vi "Sample preparation.vi"(6 "ALS mode parameter":T1={"Wash vial Location"=0.0, "Reagent volume (ul)"=[], "Reagent location"=[], "Mix vial Location"=0.0, "Pump 5 target volume (ml)"=5.0, "Pump 5  flowrate (ml/min)"=5.0, "Sample name"=""} {"Pump 5  flowrate (ml/min)" min=0.0 format="%#.4f"; "Pump 5 target volume (ml)" min=0.0 format="%#.4f"}, 7 "Syringe mode parameter":T2={"Pump 5 charge rate (ml/min)"=0.5, "Pump 5 charge volume (mL)"=0.1} {"Pump 5 charge volume (mL)" format="%#.4f"; "Pump 5 charge rate (ml/min)" format="%#.4f"}, 8 "Sample source":enum16{"Syringe", "ALS"}(ring), 9 "Experiment file path":path, 10 "Method folder":path=path "\\\\ECHEMHPLC-PC\\Chem32(2)/1/Data/OptSys.D", 11 "Configured COM ports":T3={"Pump 1 COM"="COM12", "Pump 2 COM"="COM9", "Pump 3 COM"="COM13", "Pump 4 COM"="COM4", "Pump 5 COM"="COM15"}) -> ()   [LabVIEW 2017]
uses:
  <instrlib>/Harvard Apparatus PHD Ultra Series/Harvard Apparatus PHD Ultra Series.lvlib
panel:
  out "ALS droplet time":string
  out "Pump 5 COM":refnum<visa-resource-name>="COM12"
  out "Pump 1 COM":refnum<visa-resource-name>="COM12"
  out "Pump 2 COM":refnum<visa-resource-name>="COM12"
  out "Pump 3 COM":refnum<visa-resource-name>="COM12"
  out "Pump 4 COM":refnum<visa-resource-name>="COM12"
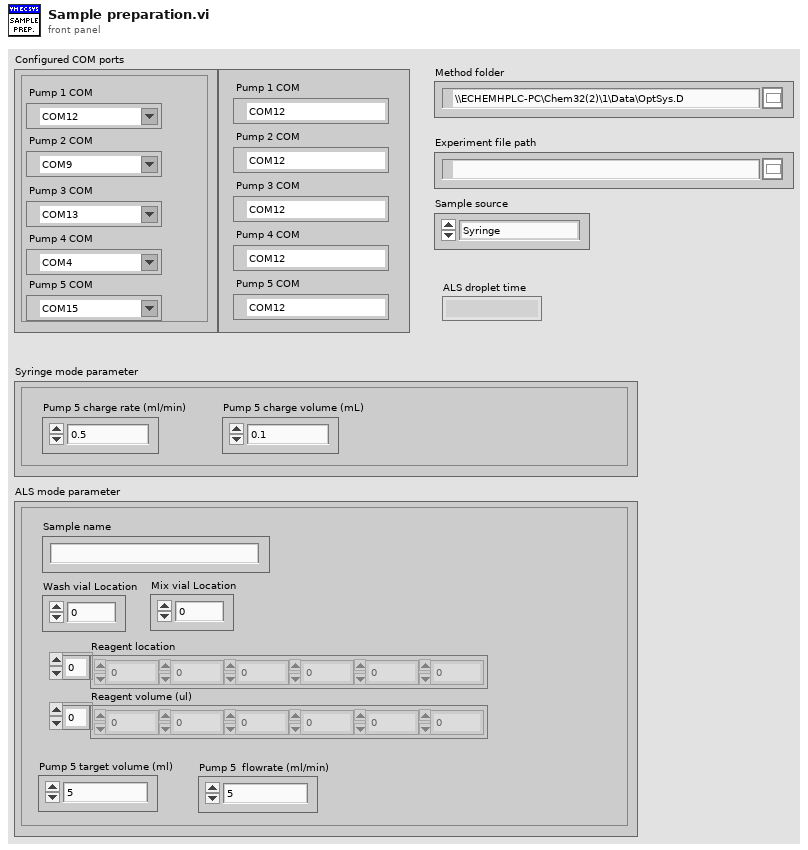
[diagram p1: front panel]
types:
  T1 = cluster{"Wash vial Location":dbl, "Reagent volume (ul)":dbl[], "Reagent location":dbl[], "Mix vial Location":dbl, "Pump 5 target volume (ml)":dbl, "Pump 5  flowrate (ml/min)":dbl, "Sample name":string}
  T2 = cluster{"Pump 5 charge rate (ml/min)":dbl, "Pump 5 charge volume (mL)":dbl}
  T3 = cluster{"Pump 1 COM":refnum<visa-resource-name>, "Pump 2 COM":refnum<visa-resource-name>, "Pump 3 COM":refnum<visa-resource-name>, "Pump 4 COM":refnum<visa-resource-name>, "Pump 5 COM":refnum<visa-resource-name>}
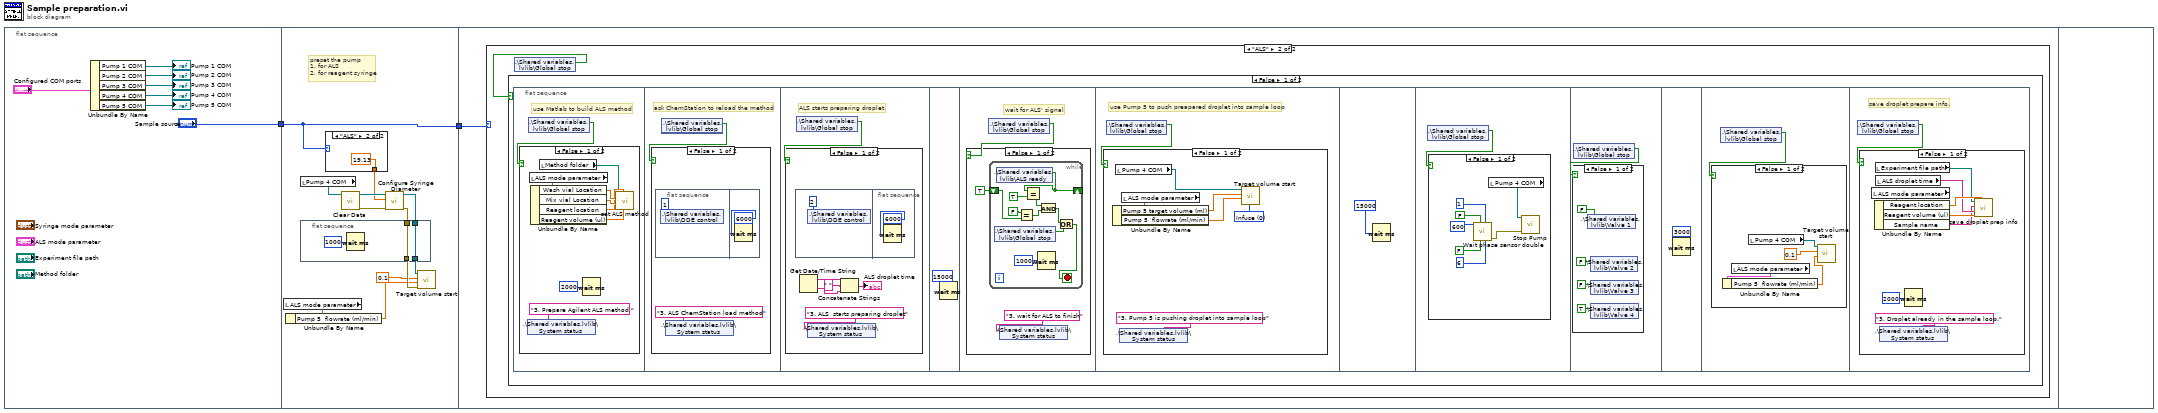
[diagram p0: block diagram]
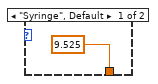
[diagram p2: hidden frame]
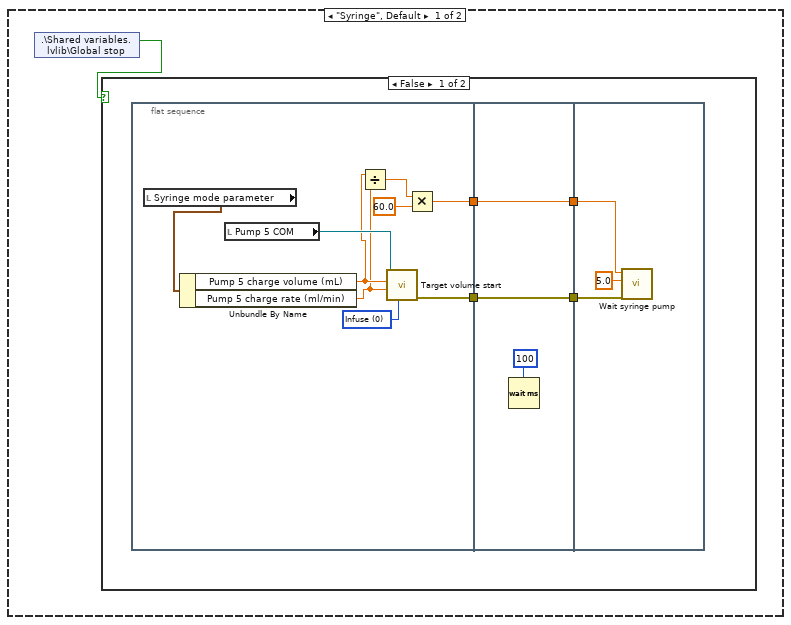
[diagram p3: hidden frame]
diagram:
  n1 = flat-sequence {
    tunnel: ["Sample source"] -> w2
    tunnel: w2 -> [w17]
    tunnel: [w17] -> w1
    tunnel: w1 -> [w27]
    frame #0 {
      n2 = Unbundle By Name("Configured COM ports") -> ("Pump 1 COM"=→"Pump 1 COM":refnum<visa-resource-name>, "Pump 2 COM"=→"Pump 2 COM":refnum<visa-resource-name>, "Pump 3 COM"=→"Pump 3 COM":refnum<visa-resource-name>, "Pump 4 COM"=→"Pump 4 COM":refnum<visa-resource-name>, "Pump 5 COM"=→"Pump 5 COM":refnum<visa-resource-name>)
    }
    frame #1 {
      # "preset the pump\n1. for ALS\n2. for reagent syringe"
      n3 = local read "ALS mode parameter"() -> (w12:T1)
      n4 = Unbundle By Name(w12) -> ("Pump 5  flowrate (ml/min)"=w11:dbl)
      n5 = local read "Pump 4 COM"() -> (w18:refnum<visa-resource-name>)
      n6 = flat-sequence {
        tunnel: [w23] -> w16
        tunnel: w15 -> [w23]
        tunnel: [w22] -> w14
        tunnel: w13 -> [w22]
        frame #0 {
          n7 = Wait (ms)(milliseconds to wait=u32 1000) -> ()  [unwired: 1 out]
        }
      }
      n8 = case shown="\"ALS\"" w17 {
        tunnel: [9.525 ("Syringe Diameter (20 mm)") 19.13 ("Syringe Diameter (20 mm)")] -> w19
        frame "Syringe", Default {
        }
        frame "ALS" {
        }
      }
      n9 = call <instrlib>:"Clear Data.vi"("VISA resource name"=w18) -> ("error out"=w21:errorcluster, "VISA resource name out"=w20:refnum<visa-resource-name>)  [unwired: 9 in]
      n10 = call <instrlib>:"Configure Syringe Diameter.vi"("error in (no error)"=w21, "Syringe Diameter (20 mm)"=w19, "VISA resource name"=w20) -> ("error out"=w15:errorcluster, "VISA resource name out"=w13:refnum<visa-resource-name>)  [unwired: 7 in]
      n11 = call "Target volume start.vi"("error in (no error)"=w16, "Flow Rate (ml/min)"=w11, "Target volume (ml)"=0.1, "VISA resource name"=w14) -> ()  [unwired: 6 in, 2 out]
    }
    frame #2 {
      n12 = case shown="\"ALS\"" w27 {
        frame "Syringe", Default {
          n13 = shared-variable ".\\Shared variables.lvlib\\Global stop"() -> (w28:bool)  [unwired: 1 in, 1 out]
          n14 = case shown="False" w28 {
            frame False {
              n15 = flat-sequence {
                tunnel: [w39] -> w32
                tunnel: [w36] -> w31
                tunnel: [w43] -> w30
                tunnel: w32 -> [w43]
                tunnel: [w42] -> w29
                tunnel: w31 -> [w42]
                tunnel: w30 -> [w47]
                tunnel: w29 -> [w45]
                frame #0 {
                  w40 = u16 0 items=["Infuse", "Withdraw"] ("Pump Direction (0:Infuse)")
                  n16 = local read "Syringe mode parameter"() -> (w35:T2)
                  n17 = Unbundle By Name(w35) -> ("Pump 5 charge volume (mL)"=w34:dbl, "Pump 5 charge rate (ml/min)"=w33:dbl)
                  n18 = local read "Pump 5 COM"() -> (w41:refnum<visa-resource-name>)
                  n19 = Divide(x=w34, y=w33) -> (x/y=w38:dbl)
                  n20 = call "Target volume start.vi"("Pump Direction (0:Infuse)"=w40, "Flow Rate (ml/min)"=w33, "Target volume (ml)"=w34, "VISA resource name"=w41) -> ("error out"=w39:errorcluster)  [unwired: 6 in, 1 out]
                  n21 = Multiply(x=w38, y=60.0) -> (x*y=w36:dbl)
                }
                frame #1 {
                  n22 = Wait (ms)(milliseconds to wait=u32 100) -> ()  [unwired: 1 out]
                }
                frame #2 {
                  n23 = call "Wait syringe pump.vi"("error in (no error)"=w47, "Delayed time (s)"=5.0, "Time Target (s)"=w45) -> ()  [unwired: 8 in, 1 out]
                }
              }
            }
            frame True {
            }
          }
        }
        frame "ALS" {
          n24 = shared-variable ".\\Shared variables.lvlib\\Global stop"() -> (w48:bool)  [unwired: 1 in, 1 out]
          n25 = case shown="False" w48 {
            frame False {
              n26 = flat-sequence {
                frame #0 {
                  # "use Matlab to build ALS method"
                  n27 = shared-variable ".\\Shared variables.lvlib\\Global stop"() -> (w49:bool)  [unwired: 1 in, 1 out]
                  n28 = case shown="False" w49 {
                    frame False {
                      n29 = shared-variable ".\\Shared variables.lvlib\\System status"("3. Prepare Agilent ALS method " ("System status")) -> ()  [unwired: 1 in, 1 out]
                      n30 = local read "ALS mode parameter"() -> (w56:T1)
                      n31 = Unbundle By Name(w56) -> ("Wash vial Location"=w55:dbl, "Mix vial Location"=w54:dbl, "Reagent location"=w52:dbl[], "Reagent volume (ul)"=w53:dbl[])
                      n32 = local read "Method folder"() -> (w51:path)
                      n33 = Wait (ms)(milliseconds to wait=u32 2000) -> ()  [unwired: 1 out]
                      n34 = call "set ALS method.vi"("Reagent volume (ul)"=w53, "Reagent location"=w52, "Mix vial Location"=w54, "Wash vial Location"=w55, "method folder"=w51) -> ()  [unwired: 7 in]
                    }
                    frame True {
                    }
                  }
                }
                frame #1 {
                  # "ask ChemStation to reload the method"
                  n35 = shared-variable ".\\Shared variables.lvlib\\Global stop"() -> (w58:bool)  [unwired: 1 in, 1 out]
                  n36 = case shown="False" w58 {
                    frame False {
                      n37 = flat-sequence {
                        frame #0 {
                          n38 = shared-variable ".\\Shared variables.lvlib\\DDE control"(i8 1 ("DDE control")) -> ()  [unwired: 1 in, 1 out]
                        }
                        frame #1 {
                          n39 = Wait (ms)(milliseconds to wait=u32 6000) -> ()  [unwired: 1 out]
                        }
                      }
                      n40 = shared-variable ".\\Shared variables.lvlib\\System status"("3. ALS ChemStation load method" ("System status")) -> ()  [unwired: 1 in, 1 out]
                    }
                    frame True {
                    }
                  }
                  n41 = shared-variable ".\\Shared variables.lvlib\\Global stop"() -> ()  [unwired: 1 in, 2 out]
                }
                frame #2 {
                  # "ALS starts preparing droplet"
                  n42 = shared-variable ".\\Shared variables.lvlib\\Global stop"() -> (w62:bool)  [unwired: 1 in, 1 out]
                  n43 = case shown="False" w62 {
                    frame False {
                      n44 = flat-sequence {
                        frame #0 {
                          n45 = shared-variable ".\\Shared variables.lvlib\\DDE control"(i8 2 ("DDE control")) -> ()  [unwired: 1 in, 1 out]
                        }
                        frame #1 {
                          n46 = Wait (ms)(milliseconds to wait=u32 6000) -> ()  [unwired: 1 out]
                        }
                      }
                      n47 = Get Date/Time String() -> (date string=w66:string, time string=w64:string)  [unwired: 3 in]
                      n48 = shared-variable ".\\Shared variables.lvlib\\System status"("3. ALS  starts preparing droplet" ("System status")) -> ()  [unwired: 1 in, 1 out]
                      n49 = Concatenate Strings(w66, " ", w64) -> (→"ALS droplet time":string)
                    }
                    frame True {
                    }
                  }
                }
                frame #3 {
                  n50 = Wait (ms)(milliseconds to wait=u32 15000) -> ()  [unwired: 1 out]
                }
                frame #4 {
                  # "wait for ALS' signal"
                  n51 = shared-variable ".\\Shared variables.lvlib\\Global stop"() -> (w71:bool)  [unwired: 1 in, 1 out]
                  n52 = case shown="False" w71 {
                    frame False {
                      n53 = while {
                        shift-right: [w80] -> _
                        shift-left: TRUE ("Boolean") -> [w79]
                        stop <- w82 stop-if-true
                        n54 = shared-variable ".\\Shared variables.lvlib\\Global stop"() -> (w83:bool)  [unwired: 1 in, 1 out]
                        n55 = shared-variable ".\\Shared variables.lvlib\\ALS ready"() -> (w80:bool)  [unwired: 1 in, 1 out]
                        n56 = Equal?(x=FALSE, y=w79) -> (x = y?=w75:bool)
                        n57 = Equal?(x=w80, y=TRUE) -> (x = y?=w76:bool)
                        n58 = Wait (ms)(milliseconds to wait=u32 1000) -> ()  [unwired: 1 out]
                        n59 = And(x=w76, y=w75) -> (x .and. y?=w74:bool)
                        n60 = Or(x=w74, y=w83) -> (x .or. y?=w82:bool)
                      }
                      n61 = shared-variable ".\\Shared variables.lvlib\\System status"("3. wait for ALS to finish" ("System status")) -> ()  [unwired: 1 in, 1 out]
                    }
                    frame True {
                    }
                  }
                }
                frame #5 {
                  # "use Pump 5 to push preapared droplet into sample loop"
                  n62 = shared-variable ".\\Shared variables.lvlib\\Global stop"() -> (w84:bool)  [unwired: 1 in, 1 out]
                  n63 = case shown="False" w84 {
                    frame False {
                      w90 = u16 0 items=["Infuse", "Withdraw"] ("Pump Direction (0:Infuse)")
                      n64 = local read "Pump 4 COM"() -> (w85:refnum<visa-resource-name>)
                      n65 = shared-variable ".\\Shared variables.lvlib\\System status"("3. Pump 5 is pushing droplet into sample loop" ("System status")) -> ()  [unwired: 1 in, 1 out]
                      n66 = local read "ALS mode parameter"() -> (w89:T1)
                      n67 = Unbundle By Name(w89) -> ("Pump 5 target volume (ml)"=w88:dbl, "Pump 5  flowrate (ml/min)"=w87:dbl)
                      n68 = call "Target volume start.vi"("Pump Direction (0:Infuse)"=w90, "Flow Rate (ml/min)"=w87, "Target volume (ml)"=w88, "VISA resource name"=w85) -> ()  [unwired: 6 in, 2 out]
                    }
                    frame True {
                    }
                  }
                }
                frame #6 {
                  n69 = Wait (ms)(milliseconds to wait=u32 15000) -> ()  [unwired: 1 out]
                }
                frame #7 {
                  n70 = shared-variable ".\\Shared variables.lvlib\\Global stop"() -> (w92:bool)  [unwired: 1 in, 1 out]
                  n71 = case shown="False" w92 {
                    frame False {
                      n72 = call "Wait phase sensor double.vi"("Phase sensor number 2"=6 ("Phase sensor number"), "Phase sensor number 1"=1 ("Phase sensor number"), "Sense 2 T/F"=FALSE ("Sense T/F"), "Sense 1 T/F"=FALSE ("Sense T/F"), "Sensitivity time (ms)"=u32 600) -> ("error IO"=w98:errorcluster)  [unwired: 6 in]
                      n73 = local read "Pump 4 COM"() -> (w99:refnum<visa-resource-name>)
                      n74 = call <instrlib>:"Stop Pump.vi"("error in (no error)"=w98, "VISA resource name"=w99) -> ()  [unwired: 8 in, 2 out]
                    }
                    frame True {
                    }
                  }
                }
                frame #8 {
                  n75 = shared-variable ".\\Shared variables.lvlib\\Global stop"() -> (w100:bool)  [unwired: 1 in, 1 out]
                  n76 = case shown="False" w100 {
                    frame False {
                      n77 = shared-variable ".\\Shared variables.lvlib\\Valve 1"(FALSE ("Valve 1")) -> ()  [unwired: 1 in, 1 out]
                      n78 = shared-variable ".\\Shared variables.lvlib\\Valve 2"(FALSE ("Valve 2")) -> ()  [unwired: 1 in, 1 out]
                      n79 = shared-variable ".\\Shared variables.lvlib\\Valve 3"(FALSE ("Valve 3")) -> ()  [unwired: 1 in, 1 out]
                      n80 = shared-variable ".\\Shared variables.lvlib\\Valve 4"(TRUE ("Valve 3")) -> ()  [unwired: 1 in, 1 out]
                    }
                    frame True {
                    }
                  }
                }
                frame #9 {
                  n81 = Wait (ms)(milliseconds to wait=u32 3000) -> ()  [unwired: 1 out]
                }
                frame #10 {
                  n82 = shared-variable ".\\Shared variables.lvlib\\Global stop"() -> (w106:bool)  [unwired: 1 in, 1 out]
                  n83 = case shown="False" w106 {
                    frame False {
                      n84 = local read "ALS mode parameter"() -> (w110:T1)
                      n85 = Unbundle By Name(w110) -> ("Pump 5  flowrate (ml/min)"=w109:dbl)
                      n86 = local read "Pump 4 COM"() -> (w107:refnum<visa-resource-name>)
                      n87 = call "Target volume start.vi"("Flow Rate (ml/min)"=w109, "Target volume (ml)"=0.1, "VISA resource name"=w107) -> ()  [unwired: 7 in, 2 out]
                    }
                    frame True {
                    }
                  }
                }
                frame #11 {
                  # "save droplet prepare info."
                  n88 = shared-variable ".\\Shared variables.lvlib\\Global stop"() -> (w111:bool)  [unwired: 1 in, 1 out]
                  n89 = case shown="False" w111 {
                    frame False {
                      n90 = local read "ALS mode parameter"() -> (w117:T1)
                      n91 = Unbundle By Name(w117) -> ("Reagent location"=w116:dbl[], "Reagent volume (ul)"=w115:dbl[], "Sample name"=w112:string)
                      n92 = local read "Experiment file path"() -> (w114:path)
                      n93 = local read "ALS droplet time"() -> (w113:string)
                      n94 = shared-variable ".\\Shared variables.lvlib\\System status"("3. Droplet already in the sample loop." ("System status")) -> ()  [unwired: 1 in, 1 out]
                      n95 = Wait (ms)(milliseconds to wait=u32 2000) -> ()  [unwired: 1 out]
                      n96 = call "save droplet prep info.vi"("Reagent volume (ul)"=w115, "Reagent location"=w116, "Sample preparation time"=w113, "Sample name"=w112, "Exp. file path"=w114) -> ()  [unwired: 7 in]
                    }
                    frame True {
                    }
                  }
                }
              }
            }
            frame True {
            }
          }
        }
      }
    }
    frame #3 {
    }
  }
